vi "Main RT.vi"() -> ()   [LabVIEW 2013]
uses:
  Globals - Monitoring Variables.vi
  Globals - UI and RT Streams.vi
  Global - Configuration.vi
panel:
  in  "Acq and Logging Props":T1
  in  "Message Cluster":cluster{"Message":string, "Value":variant}
  in  "Log (current)\nFile Reference":refnum<k34>
  in  "Acq and Log Queue":refnum<queue>
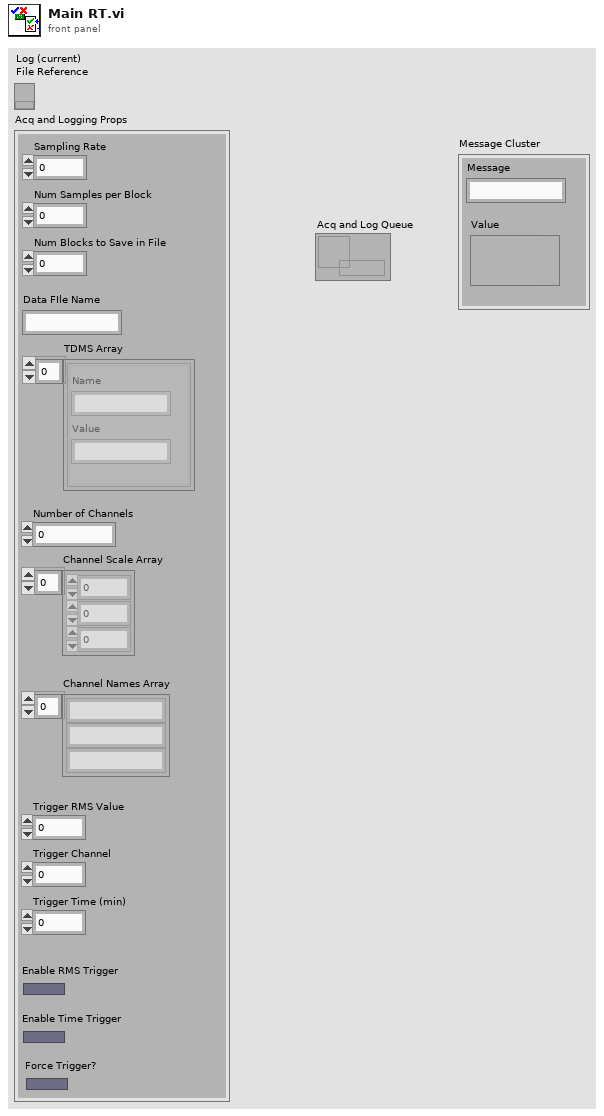
[diagram p1: front panel]
types:
  T1 = cluster{"Sampling Rate":dbl, "Num Samples per Block":i32, "Num Blocks to Save in File":i32, "Data FIle Name":string, "TDMS Array":cluster{"Name":string, "Value":string}[], "Number of Channels":i32, "Channel Scale Array":dbl[], "Channel Names Array":string[], "Trigger RMS Value":dbl, "Trigger Channel":i32, "Trigger Time (min)":i32, "Enable RMS Trigger":bool, "Enable Time Trigger":bool, "Force Trigger?":bool}
  T2 = cluster{"Sampling Rate":dbl, "Num Samples per Block":i32, "Num Blocks to Save in File":i32, "Data FIle Name":string, "TDMS Array":cluster{"Name":string, "Value":string}[], "Number of Channels":i32, "Channel Scale Array":dbl[], "Channel Names Array":string[], "Trigger RMS Value":dbl, "Trigger Channel":i32, "Trigger Time (min)":i32, "Enable RMS Trigger":bool, "Enable Time Trigger":bool, "Always Log":bool}
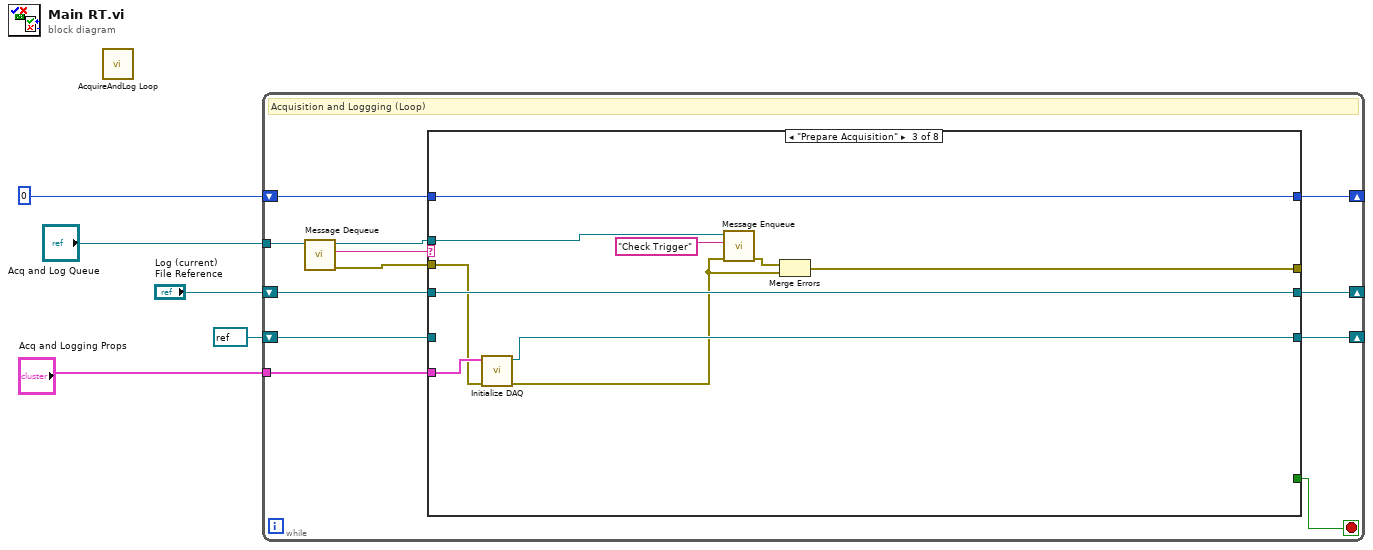
[diagram p0: block diagram]
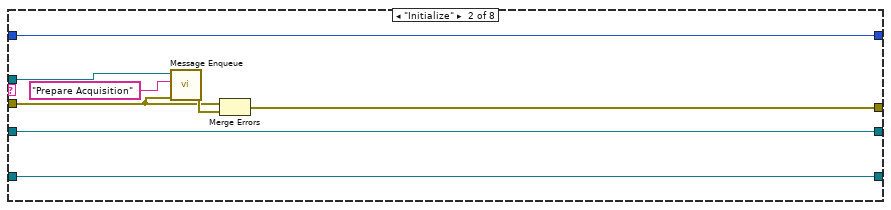
[diagram p3: hidden frame]
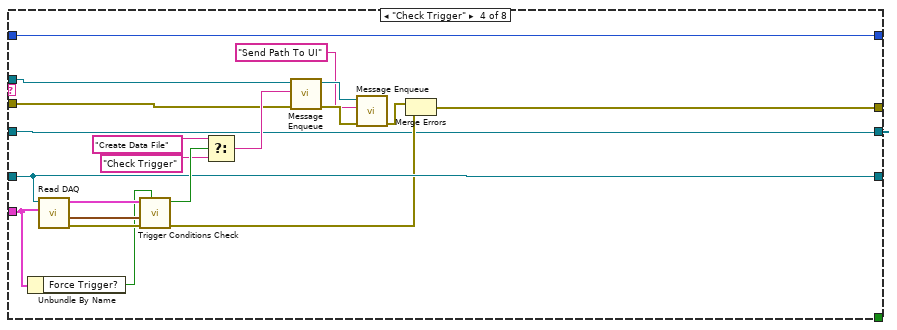
[diagram p4: hidden frame]
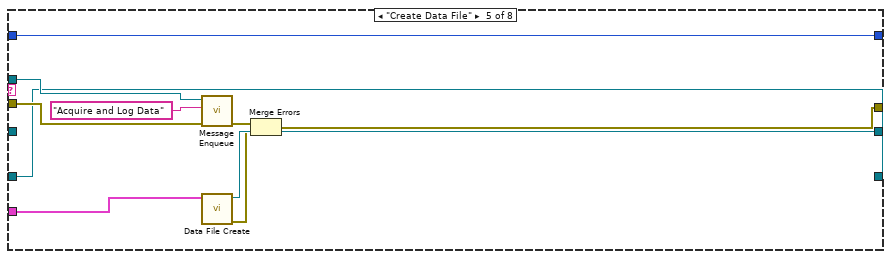
[diagram p5: hidden frame]
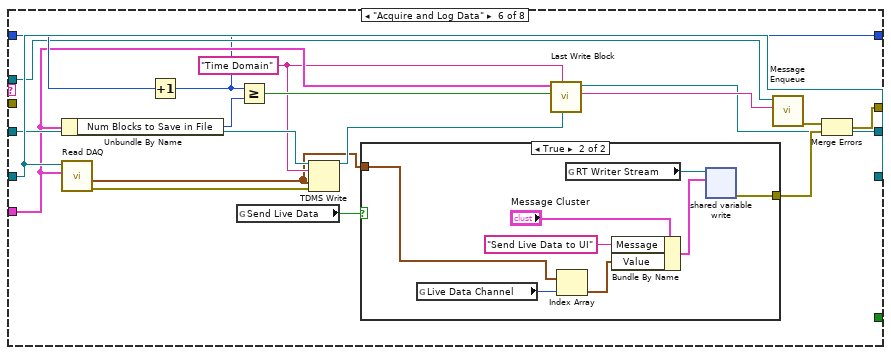
[diagram p6: hidden frame]
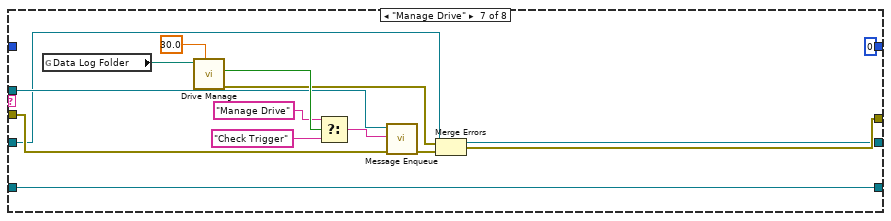
[diagram p8: hidden frame]
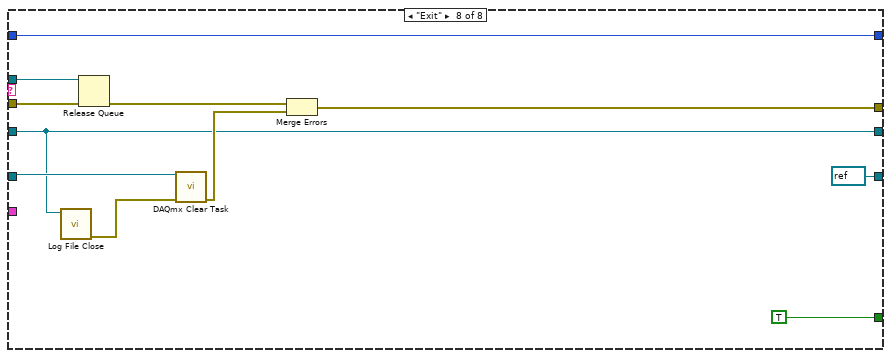
[diagram p9: hidden frame]
diagram:
  n1 = call "AcquireAndLog Loop.vi"() -> ()  [unwired: 12 in]
  n2 = while {
    tunnel: "Acq and Log Queue" -> [w16]
    tunnel: "Acq and Logging Props" -> [w13]
    shift-right: [w12] -> _
    shift-left: refnum<k21> refnum ("DAQmx Task Name") -> [w11]
    shift-right: [w10] -> _
    shift-left: "Log (current)\nFile Reference" -> [w9]
    shift-right: [w7] -> _
    shift-left: 0 -> [w8]
    stop <- w6 stop-if-true
    # "Acquisition and Loggging (Loop)"
    n3 = call "Message Dequeue.vi"("Message Queue"=w16) -> ("error out"=w14:errorcluster, "Message"=w17:string, "Message Queue dup"=w15:refnum<queue>)  [unwired: 5 in, 1 out]
    n4 = case shown="\"Prepare Acquisition\"" w17 {
      tunnel: w15 -> [_ w29 w36 w56 w67 w80 w102 w117]
      tunnel: w14 -> [w18 w26 w30 w50 w65 _ w101 w116]
      tunnel: [w18 w25 w34 w49 w64 w71 w99 w112] -> _
      tunnel: w13 -> [_ _ w38 w40 w59 w78 _ _]
      tunnel: [w19 w24 w37 w51 w63 w86 w95 refnum<k21> refnum ("DAQmx Task Name")] -> w12
      tunnel: w11 -> [w19 w24 _ w51 w63 w86 w95 w119]
      tunnel: [w20 w23 w33 w42 w68 w69 w96 w111] -> w10
      tunnel: w9 -> [w20 w23 w33 w42 _ w85 w96 w111]
      tunnel: w8 -> [w21 w22 w32 w43 w60 w83 _ w109]
      tunnel: [w21 w22 w32 w43 w60 w70 0 w109] -> w7
      tunnel: [_ _ _ _ _ _ _ TRUE] -> w6
      frame "False", Default {
      }
      frame "Initialize" {
        n5 = call "Message Enqueue.vi"("error in (no error)"=w26, "Message"="Prepare Acquisition", "Message Queue"=w29) -> ("error out"=w27:errorcluster)  [unwired: 7 in, 1 out]
        n6 = Merge Errors(w26, w27) -> (w25:errorcluster)
      }
      frame "Prepare Acquisition" {
        n7 = call "Initialize DAQ.vi"("error in (no error)"=w30, "Acq and Logging Props"=w38) -> ("DAQmx Task Name"=w37:refnum<k21>)  [unwired: 8 in, 1 out]
        n8 = call "Message Enqueue.vi"("error in (no error)"=w30, "Message"="Check Trigger", "Message Queue"=w36) -> ("error out"=w31:errorcluster)  [unwired: 7 in, 1 out]
        n9 = Merge Errors(w31, w30) -> (w34:errorcluster)
      }
      frame "Check Trigger" {
        n10 = Unbundle By Name(w40) -> ("Force Trigger?"=w39:bool)
        n11 = call "Read DAQ.vi"("Acq and Logging Props"=w40, "DAQmx Task Name"=w51) -> ("error out"=w57:errorcluster, "Waveform Data"=w58:waveform(dbl)[], "Acq and Logging Props dup"=w41:T2)  [unwired: 7 in]
        n12 = call "Trigger Conditions Check.vi"("Force Trigger?"=w39, "error in (no error)"=w57, "Waveform Data"=w58, "Acq and Logging Props"=w41) -> ("error out"=w48:errorcluster, "Trigger Condition Met?"=w55:bool)  [unwired: 6 in]
        n13 = Select(t="Create Data File", s=w55, f="Check Trigger") -> (s? t:f=w52:string)
        n14 = call "Message Enqueue.vi"("error in (no error)"=w50, "Message"=w52, "Message Queue"=w56) -> ("error out"=w46:errorcluster, "Message Queue dup"=w47:refnum<queue>)  [unwired: 7 in]
        n15 = call "Message Enqueue.vi"("error in (no error)"=w46, "Message"="Send Path To UI", "Message Queue"=w47) -> ("error out"=w44:errorcluster)  [unwired: 7 in, 1 out]
        n16 = Merge Errors(w44, w48) -> (w49:errorcluster)
      }
      frame "Create Data File" {
        n17 = call "Message Enqueue.vi"("error in (no error)"=w65, "Message"="Acquire and Log Data", "Message Queue"=w67) -> ("error out"=w62:errorcluster)  [unwired: 7 in, 1 out]
        n18 = call "Data File Create.vi"("Acq and Logging Props"=w59) -> ("error out"=w61:errorcluster, "TDMS File Reference"=w68:refnum<k34>)  [unwired: 9 in]
        n19 = Merge Errors(w62, w61) -> (w64:errorcluster)
      }
      frame "Acquire and Log Data" {
        w77 = "Time Domain" ("group name in (Untitled)")
        n20 = Unbundle By Name(w78) -> ("Num Blocks to Save in File"=w82:i32)
        n21 = call "Read DAQ.vi"("Acq and Logging Props"=w78, "DAQmx Task Name"=w86) -> ("error out"=w84:errorcluster, "Waveform Data"=w74:waveform(dbl)[])  [unwired: 7 in, 1 out]
        n22 = Increment(x=w83) -> (x+1=w70:i32)
        n23 = global read "Globals - Monitoring Variables.vi" "Send Live Data"() -> (w81:bool)
        n24 = Greater Or Equal?(x=w70, y=w82) -> (x >= y?=w79:bool)
        n25 = TDMS Write(0:w85, 5:w77, 9:w74, 11:w84) -> (4:w75:refnum<k34>)  [unwired: 2 in, 3 out]
        n26 = case shown="True" w81 {
          tunnel: w74 -> [_ w93]
          tunnel: [_ w87] -> w72
          frame False {
          }
          frame True {
            n27 = global read "Globals - Monitoring Variables.vi" "Live Data Channel"() -> (w94:u32)
            n28 = Index Array(array=w93, index=w94) -> (element=w91:waveform(dbl))
            n29 = global read "Globals - UI and RT Streams.vi" "RT Writer Stream"() -> (w88:refnum<k21>)
            n30 = Bundle By Name(cluster="Message Cluster", "Message"="Send Live Data to UI", "Value"=w91) -> (w89:cluster{"Message":string, "Value":variant})
            n31 = shared-variable-write(w88, w89) -> (w87:errorcluster)  [unwired: 2 in, 2 out]
          }
        }
        n32 = call "Last Write Block.vi"("tdms file Ref"=w75, "Group Name TMDS"=w77, "End Block?"=w79, "Acq and Logging Props"=w78) -> ("Message"=w76:string, "tdms file out"=w69:refnum<k34>)  [unwired: 5 in, 1 out]
        n33 = call "Message Enqueue.vi"("Message"=w76, "Message Queue"=w80) -> ("error out"=w73:errorcluster)  [unwired: 8 in, 1 out]
        n34 = Merge Errors(w73, w72) -> (w71:errorcluster)
      }
      frame "Manage Drive" {
        n35 = global read "Global - Configuration.vi" "Data Log Folder"() -> (w108:path)
        n36 = call "Drive Manage.vi"("Min Drive Free Space (%)"=30.0, "Data Folder"=w108) -> ("error out"=w98:errorcluster, "Drive Space Below Limit"=w106:bool)  [unwired: 8 in]
        n37 = Select(t="Manage Drive", s=w106, f="Check Trigger") -> (s? t:f=w103:string)
        n38 = call "Message Enqueue.vi"("error in (no error)"=w101, "Message"=w103, "Message Queue"=w102) -> ("error out"=w97:errorcluster)  [unwired: 7 in, 1 out]
        n39 = Merge Errors(w98, w97) -> (w99:errorcluster)
      }
      frame "Exit" {
        n40 = call "Log File Close.vi"("Log File"=w111) -> ("error out"=w115:errorcluster)  [unwired: 10 in]
        n41 = Release Queue(queue=w117, error in (no error)=w116) -> (error out=w114:errorcluster)  [unwired: 1 in, 2 out]
        n42 = call <vilib>:"DAQmx Clear Task.vi"("task in"=w119, "error in"=w115) -> ("error out"=w113:errorcluster)  [unwired: 13 in]
        n43 = Merge Errors(w114, w113) -> (w112:errorcluster)
      }
    }
  }
